vi "TwoPointCaculateAngle.vi"(2 "Point2":cluster{"X":dbl, "Y":dbl}, 3 "Point1":cluster{"X":dbl, "Y":dbl}) -> (0 "角度":dbl)   [LabVIEW 2014]
uses:
  <vilib>/vision/NI_Vision_Development_Module.lvlib
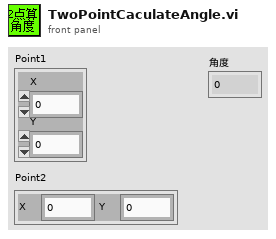
[diagram p1: front panel]
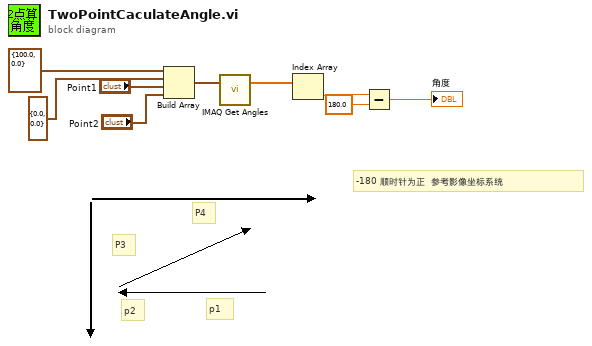
[diagram p0: block diagram]
diagram:
  # "-180 顺时针为正  参考影像坐标系统"
  # "P4"
  # "P3"
  # "p1"
  # "p2"
  n1 = Build Array(cluster{"X":dbl, "Y":dbl} {"X"=100.0, "Y"=0.0} ("element"), cluster{"X":dbl, "Y":dbl} {"X"=0.0, "Y"=0.0} ("element"), "Point1", "Point2") -> (w9:cluster{"X":dbl, "Y":dbl}[])
  n2 = call "IMAQ Get Angles"("Points"=w9) -> ("Angles (deg)"=w8:sgl[])  [unwired: 4 in, 2 out]
  n3 = Index Array(array=w8) -> (element=w3:sgl)  [unwired: 1 in]
  n4 = Subtract(x=w3, y=sgl 180.0) -> (x-y=→"角度":sgl)
